vi "动态反馈数据-1.vi"(11 "数组":u8[](array[numeric])) -> (2 "修正值":T1, 3 "飞机安装-识别码":string caption="识别码")   [LabVIEW 2012]
uses:
  index-i8.vi
  index-i16.vi
  XX-I16.vi
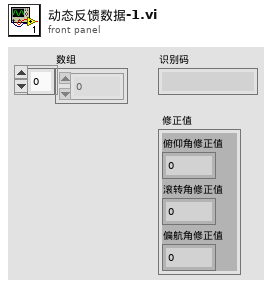
[diagram p1: front panel]
types:
  T1 = cluster{"俯仰角修正值":i16, "滚转角修正值":i16, "偏航角修正值":i16}
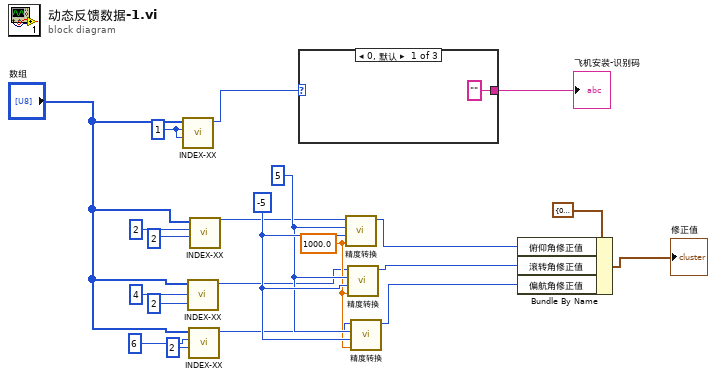
[diagram p0: block diagram]
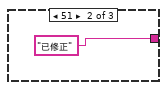
[diagram p2: hidden frame]
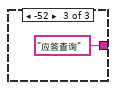
[diagram p3: hidden frame]
diagram:
  w19 = 1 ("索引")
  w15 = i16 -5 ("下限")
  w14 = i16 5 ("上限")
  w13 = 1000.0 ("单位")
  n1 = call-poly "INDEX-XX.vi"("长度"=w19, "索引"=w19, "数组"="数组") -> ("数值输出"=w20:i8)  [unwired: 8 in]
  n2 = call-poly "INDEX-XX.vi"("长度"=2, "索引"=4, "数组"="数组") -> ("数值输出"=w4:i16)  [unwired: 8 in]
  n3 = call-poly "INDEX-XX.vi"("长度"=2, "索引"=6, "数组"="数组") -> ("数值输出"=w3:i16)  [unwired: 8 in]
  n4 = call-poly "INDEX-XX.vi"("长度"=2, "索引"=2, "数组"="数组") -> ("数值输出"=w6:i16)  [unwired: 8 in]
  n5 = case shown="0, 默认" w20 {
    tunnel: ["" ("字符串") "已修正" ("字符串") "应答查询" ("字符串")] -> w21
    frame 0, Default {
    }
    frame 51 {
    }
    frame -52 {
    }
  }
  "飞机安装-识别码" <- w21
  n6 = call-poly "精度转换.vi"("单位"=w13, "下限"=w15, "上限"=w14, "数值输入"=w6) -> ("输出"=w5:i16)  [unwired: 7 in]
  n7 = call-poly "精度转换.vi"("单位"=w13, "下限"=w15, "上限"=w14, "数值输入"=w4) -> ("输出"=w2:i16)  [unwired: 7 in]
  n8 = call-poly "精度转换.vi"("单位"=w13, "下限"=w15, "上限"=w14, "数值输入"=w3) -> ("输出"=w1:i16)  [unwired: 7 in]
  n9 = Bundle By Name(cluster=T1 {"俯仰角修正值"=0, "滚转角修正值"=0, "偏航角修正值"=0} ("修正值"), "俯仰角修正值"=w5, "滚转角修正值"=w2, "偏航角修正值"=w1) -> (→"修正值":T1)
